vi "利用勾股定理求直角三角形斜边.vi"(1 "b":dbl=4.0, 2 "a":dbl=3.0) -> (0 "c":dbl=5.0)   [LabVIEW 2012, in "几何工具.lvlib"]
doc: "功能：\n\n利用勾股定理计算直角三角形斜边的长度。\n\n公式：\n\nc=sqrt(a^2+b^2)"
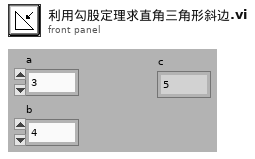
[diagram p1: front panel]
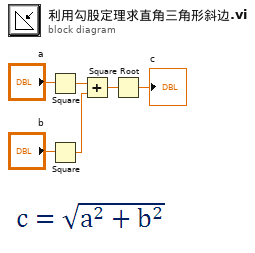
[diagram p0: block diagram]
diagram:
  n1 = Square(x="a") -> (x^2=w4:dbl)
  n2 = Square(x="b") -> (x^2=w3:dbl)
  n3 = Add(x=w4, y=w3) -> (x+y=w2:dbl)
  n4 = Square Root(x=w2) -> (sqrt(x)=→"c":dbl)
